vi "VideoTomv3.vi"() -> ()   [LabVIEW 2016]
uses:
  <vilib>/Utility/file.llb/Write Delimited Spreadsheet (DBL).vi
  <vilib>/vision/NI_Vision_Development_Module.lvlib
panel:
  in  "Skip First n Particles":i32
  in  "Exclusion\nFraction":dbl=0.2
  out "Total Frames":i32
  out "Frame No":dbl
  in  "Max Displ.":dbl=10.0
  in  "Max Frame Jump":i8=3
  out "FPS":i32
  out "Particle Image":T1(plugin-control)
  in  "Match Parameters":T2={"Number of Matches Requested"=500, "Minimum Match Score"=750.0, "Angle Ranges"=[]} {"Angle Ranges"."End Angle" min=-360 max=360; "Angle Ranges"."Start Angle" min=-360 max=360; "Minimum Match Score" min=0 max=1000; "Number of Matches Requested" min=1 max=9999}
  out "Current File Root":string
  in  "Video Folder Path":path=path "C:/Users/TomDixon/Desktop/170404"
  in  "Vids Per Particle":i32=1
  in  "Particles":i32=1
  # "Exclusion Fraction is the fraction of the image auto-excluded from masking\nSet as high as you can without error!"
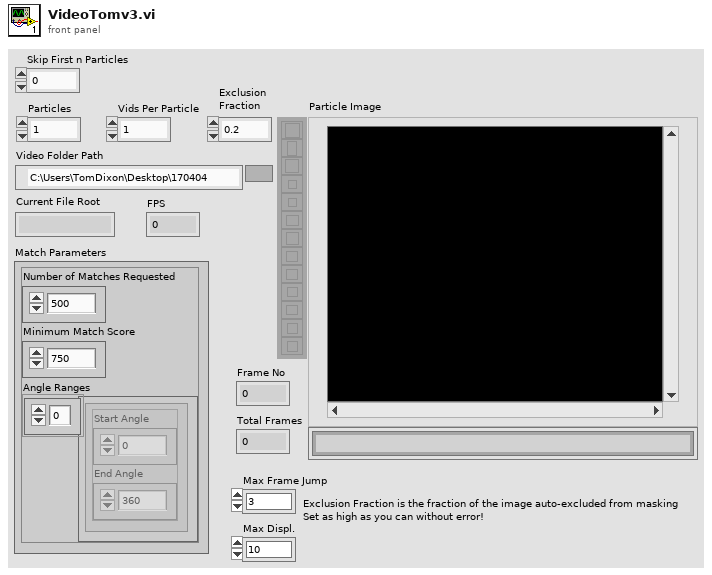
[diagram p1: front panel]
types:
  T1 = typedef "IMAQ Image.ctl" = refnum<image>
  T2 = cluster{"Number of Matches Requested":i32, "Minimum Match Score":sgl, "Angle Ranges":cluster{"Start Angle":sgl, "End Angle":sgl}[]}
  T3 = typedef "AviRefnum.ctl" = refnum<k1>
  T4 = typedef "Image Type" = u32
  T5 = cluster{"width":u32, "height":u32, "framesPerSecond":u32, "compressionFilter":string, "hasData":bool}
  T6 = cluster{"Position":cluster{"x":sgl, "y":sgl}, "Angle":sgl, "Scale":sgl, "Score":sgl, "Bounding Box":cluster{"x":sgl, "y":sgl}[]}[]
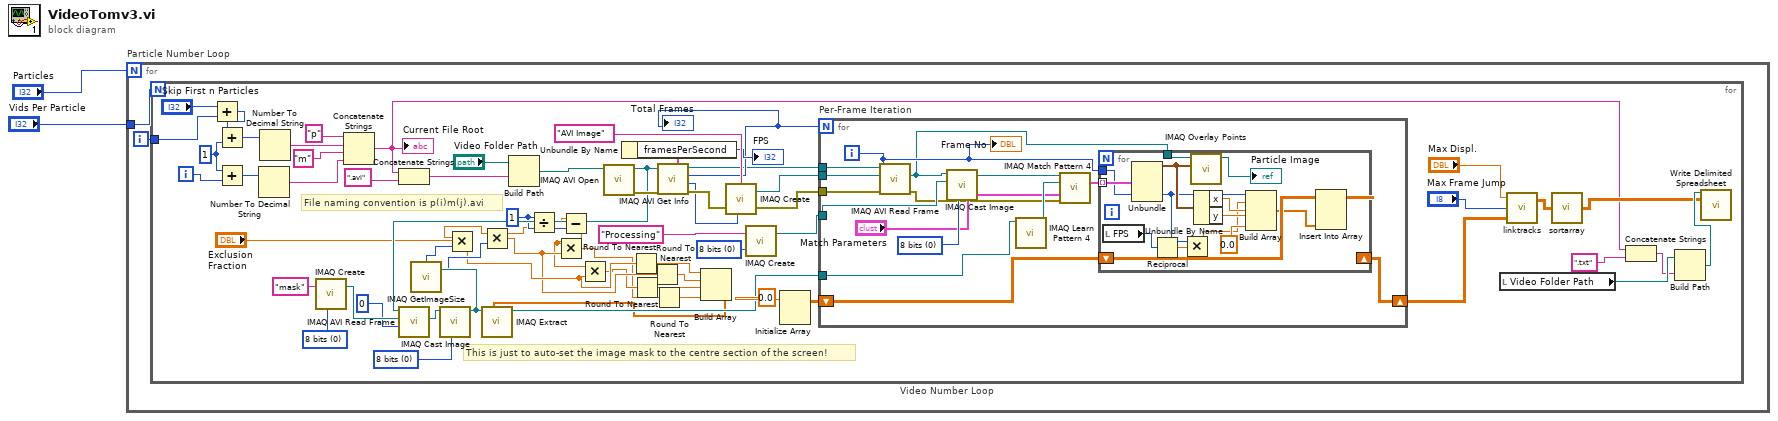
[diagram p0: block diagram]
diagram:
  n1 = for "Particle Number Loop" {
    N: "Particles" -> [_]
    tunnel: "Vids Per Particle" -> [w4]
    i -> [w3]
    n2 = for "Video Number Loop" {
      N: w4 -> [_]
      tunnel: w3 -> [w6]
      i -> [w59]
      w10 = 1
      w27 = u32 0 items=["8 bits", "16 bits", "Float", "Complex", "RGB", "HSL"] ("Image Type")
      w36 = u32 0 items=["8 bits", "16 bits", "Float", "Complex", "RGB", "HSL"] ("Image Type")
      w39 = u32 0 items=["8 bits", "16 bits", "Float", "Complex", "RGB", "HSL"] ("Image Type")
      w60 = 1
      # "This is just to auto-set the image mask to the centre section of the screen!"
      # "File naming convention is p(i)m(j).avi"
      n3 = Add(x="Skip First n Particles", y=w6) -> (x+y=w5:i32)
      n4 = Add(x=w5, y=w60) -> (x+y=w61:i32)
      n5 = Add(x=w60, y=w59) -> (x+y=w58:i32)
      n6 = Number To Decimal String(number=w58) -> (decimal integer string=w65:string)  [unwired: 1 in]
      n7 = Number To Decimal String(number=w61) -> (decimal integer string=w67:string)  [unwired: 1 in]
      n8 = call "IMAQ Create"("Image Name"="mask", "Image Type"=w39) -> ("New Image"=w29:T1)  [unwired: 3 in, 1 out]
      n9 = Concatenate Strings("p", w67, "m", w65) -> (w24:string)
      "Current File Root" <- w24
      n10 = Concatenate Strings(w24, ".avi") -> (w62:string)
      n11 = Build Path(base path="Video Folder Path", name or relative path=w62) -> (appended path=w47:path)
      n12 = Divide(x=w10, y="Exclusion\nFraction") -> (x/y=w11:dbl)
      n13 = Subtract(x=w11, y=w10) -> (x-y=w9:dbl)
      n14 = call "IMAQ AVI Open"("AVI Path"=w47) -> ("error out"=w57:errorcluster, "Avi Refnum"=w30:T3)  [unwired: 9 in]
      n15 = call "IMAQ AVI Read Frame"("Frame Number"=u16 0, "Image"=w29, "Avi Refnum"=w30) -> ("Image Out"=w28:T1)  [unwired: 5 in, 3 out]
      n16 = call "IMAQ Cast Image"("Image Type"=w27, "Image Src"=w28) -> ("Image Dst Out"=w23:T1)  [unwired: 8 in, 1 out]
      n17 = call "IMAQ GetImageSize"("Image"=w23) -> ("Y Resolution"=w21:i32, "X Resolution"=w22:i32)  [unwired: 3 in, 1 out]
      n18 = Multiply(x="Exclusion\nFraction", y=w22) -> (x*y=w15:dbl)
      n19 = Multiply(x="Exclusion\nFraction", y=w21) -> (x*y=w14:dbl)
      n20 = Multiply(x=w9, y=w14) -> (x*y=w12:dbl)
      n21 = Multiply(x=w9, y=w15) -> (x*y=w13:dbl)
      n22 = Round To Nearest(number=w15) -> (nearest integer value=w20:dbl)
      n23 = Round To Nearest(number=w13) -> (nearest integer value=w18:dbl)
      n24 = Round To Nearest(number=w14) -> (nearest integer value=w19:dbl)
      n25 = Round To Nearest(number=w12) -> (nearest integer value=w17:dbl)
      n26 = call "IMAQ AVI Get Info"("error in (no error)"=w57, "Avi Refnum"=w30) -> ("error out"=w55:errorcluster, "Image Type"=w53:T4, "Number of Frames"=w37:u32, "Avi Refnum (duplicate)"=w31:T3, "Frame Data"=w56:T5)  [unwired: 5 in]
      "Total Frames" <- w37
      n27 = Unbundle By Name(w56) -> ("framesPerSecond"=→"FPS":u32)
      n28 = Build Array(w20, w19, w18, w17) -> (w16:dbl[])
      n29 = call "IMAQ Extract"("Optional Rectangle"=w16, "Image Src"=w23) -> ("Image Dst Out"=w26:T1)  [unwired: 8 in, 1 out]
      n30 = call "IMAQ Create"("Image Name"="AVI Image", "Image Type"=w53, "error in (no error)"=w55) -> ("New Image"=w52:T1, "error out"=w51:errorcluster)  [unwired: 2 in]
      n31 = call "IMAQ Create"("Image Name"="Processing", "Image Type"=w36) -> ("New Image"=w34:T1)  [unwired: 3 in, 1 out]
      n32 = Initialize Array(0.0 ("element")) -> (w48:dbl[][])  [unwired: 2 in]
      n33 = for "Per-Frame Iteration" {
        N: w37 -> [_]
        tunnel: w31 -> [w83]
        tunnel: w52 -> [w82]
        tunnel: w51 -> [w81]
        shift-right: [w79] -> w33
        shift-left: w48 -> [w80]
        tunnel: w34 -> [w75]
        tunnel: w26 -> [w69]
        i -> [w78]
        w77 = u32 0 items=["8 bits", "16 bits", "Float", "Complex", "RGB", "HSL"] ("Image Type")
        n34 = call "IMAQ AVI Read Frame"("error in (no error)"=w81, "Frame Number"=w78, "Image"=w82, "Avi Refnum"=w83) -> ("error out"=w70:errorcluster, "Image Out"=w76:T1)  [unwired: 4 in, 2 out]
        n35 = call "IMAQ Cast Image"("Image Type"=w77, "Image Dst"=w75, "Image Src"=w76) -> ("Image Dst Out"=w74:T1)  [unwired: 7 in, 1 out]
        n36 = call "IMAQ Learn Pattern 4"("Image"=w69) -> ("Template Image Out"=w73:T1)  [unwired: 8 in, 2 out]
        n37 = call "IMAQ Match Pattern 4"("Image"=w74, "Template Image"=w73, "Parameters"="Match Parameters", "error in (no error)"=w70) -> ("Matches (pixel)"=w72:T6)  [unwired: 7 in, 4 out]
        n38 = for {
          tunnel: w72 -> [w97] mode=indexing
          tunnel: w76 -> [w96]
          tunnel: w78 -> [w90]
          shift-right: [w86] -> w79
          shift-left: w80 -> [w88]
          n39 = local read "FPS"() -> (w84:i32)
          n40 = Unbundle(w97) -> ("Position"=w94:cluster{"x":sgl, "y":sgl})  [unwired: 4 out]
          n41 = Reciprocal(x=w84) -> (1/x=w85:dbl)
          n42 = Multiply(x=w90, y=w85) -> (x*y=w89:dbl)
          n43 = call "IMAQ Overlay Points"("Point"=w94, "Image"=w96) -> ("Image Out"=→"Particle Image":T1)  [unwired: 8 in, 1 out]
          n44 = Unbundle By Name(w94) -> ("x"=w91:sgl, "y"=w92:sgl)
          n45 = Build Array(w90, w89, w91, w92, 0.0 ("element")) -> (w87:dbl[])
          n46 = Insert Into Array(array=w88, new element=w87) -> (w86:dbl[][])  [unwired: 2 in]
        }
        "Frame No" <- w78
      }
      n47 = local read "Video Folder Path"() -> (w42:path)
      n48 = call "linktracks.vi"("all rows 2"=w33, "maximum frame jump"="Max Frame Jump", "maximum displacement"="Max Displ.") -> ("all rows"=w44:sgl[][])  [unwired: 1 out]
      n49 = call "sortarray.vi"("all rows"=w44) -> ("2D data"=w32:sgl[][])
      n50 = Concatenate Strings(w24, ".txt") -> (w41:string)
      n51 = Build Path(base path=w42, name or relative path=w41) -> (appended path=w40:path)
      n52 = call-poly <vilib>:"Write Delimited Spreadsheet.vi"("file path (dialog if empty)"=w40, "2D data"=w32) -> ()  [unwired: 12 in, 2 out]
    }
  }
